vi "Config Analog Outputs.vi"(0 "VISA resource name":refnum<visa-resource-name>, 1 "High Value (0.0000)":dbl min=-1000.0 max=1000.0 step=0.0001 format="%.4f", 2 "Low Value (0.0000)":dbl min=-1000.0 max=1000.0 step=0.0001 format="%.4f", 3 "Manual Value (0.00)":dbl min=-100.0 max=100.0 step=0.01 format="%.2f", 5 "Analog Output (0: 1)":u16(ring) items=["1", "2"], 7 "Bipolar Enable (F: Bipolar Disable)":bool, 9 "Analog Output\nMode (0: Off)":u16(ring) items=["Off", "Input", "Manual", "Loop"], 11 "error in (no error)":errorcluster, 12 "Input to Monitor (0: A)":u16(ring) items=["A", "B", "C", "D"], 13 "Input Source (0: Kelvin)":u16(ring) items=["Kelvin", "Celsius", "Sensor Units", "Linear Equation"]) -> (4 "VISA resource name out":refnum<visa-resource-name>, 15 "error out":errorcluster)   [LabVIEW 2024, in "Lake Shore Cryotronics 340.lvlib"]
doc: "This VI Configures the parameters of the analog outputs."
uses:
  Lake Shore Cryotronics 340.lvlib
panel:
  # "Bipolar Enable\nBipolar Disable"
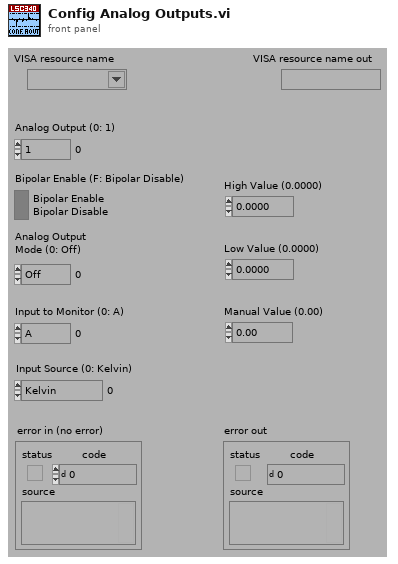
[diagram p1: front panel]
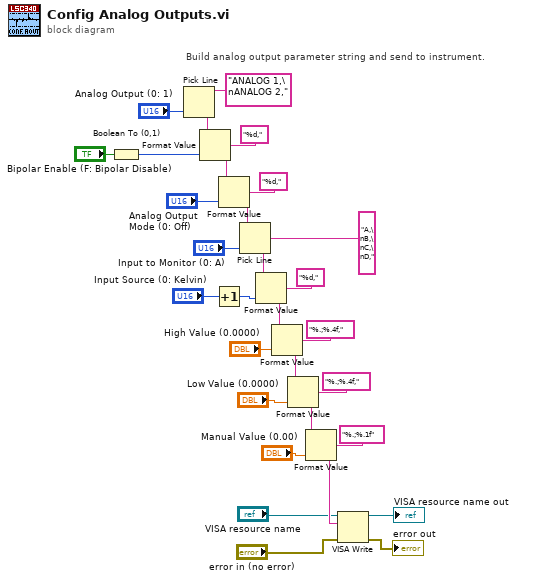
[diagram p0: block diagram]
diagram:
  # "Build analog output parameter string and send to instrument."
  n1 = Boolean To (0,1)(Boolean="Bipolar Enable (F: Bipolar Disable)") -> (0, 1=w23:i16)
  n2 = Pick Line(multi-line string="ANALOG 1,\nANALOG 2,", line index="Analog Output (0: 1)") -> (output string=w16:string)  [unwired: 1 in]
  n3 = Format Value(string ("")=w16, format string="%d,", value (0)=w23) -> (output string=w14:string)
  n4 = Increment(x="Input Source (0: Kelvin)") -> (x+1=w18:u16)
  n5 = Format Value(string ("")=w14, format string="%d,", value (0)="Analog Output\nMode (0: Off)") -> (output string=w25:string)
  n6 = Pick Line(string ("")=w25, multi-line string="A,\nB,\nC,\nD,", line index="Input to Monitor (0: A)") -> (output string=w28:string)
  n7 = Format Value(string ("")=w28, format string="%d,", value (0)=w18) -> (output string=w12:string)
  n8 = Format Value(string ("")=w12, format string="%.;%.4f,", value (0)="High Value (0.0000)") -> (output string=w1:string)
  n9 = Format Value(string ("")=w1, format string="%.;%.4f,", value (0)="Low Value (0.0000)") -> (output string=w6:string)
  n10 = Format Value(string ("")=w6, format string="%.;%.1f", value (0)="Manual Value (0.00)") -> (output string=w11:string)
  n11 = VISA Write(VISA resource name="VISA resource name", write buffer=w11, error in (no error)="error in (no error)") -> (VISA resource name out=→"VISA resource name out":refnum<visa-resource-name>, error out=→"error out":errorcluster)  [unwired: 1 out]
